vi "handshake_end.vi"(8 "error in (no error)":errorcluster, 11 "server_response (json)":string) -> (0 "error out":errorcluster, 3 "authentication":string)   [LabVIEW 2017, in "rethinkdb.lvlib"]
uses:
  rethinkdb.lvlib
  d907db94-4fb8-4ff2-8f9c-6f68c4a03077.vi
  json_get_names.vi
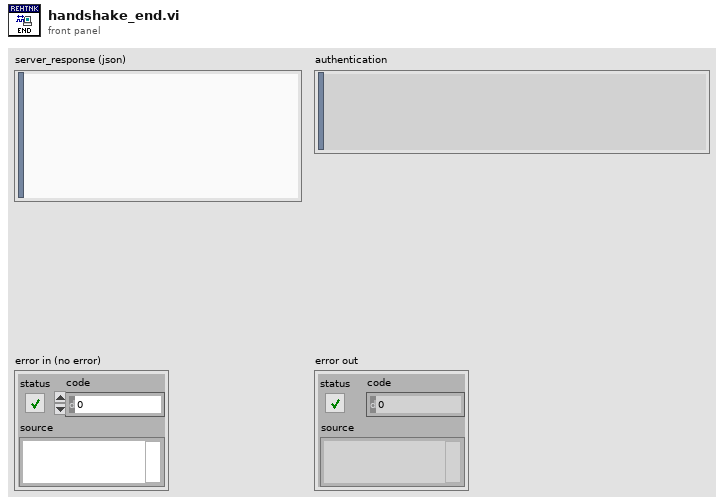
[diagram p1: front panel]
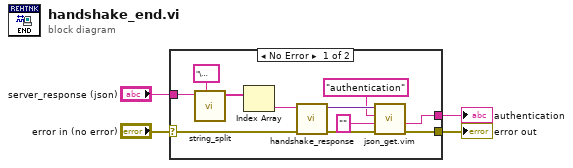
[diagram p0: block diagram]
diagram:
  n1 = case shown="No Error" "error in (no error)" {
    selector: "error in (no error)" -> [w12 w16]
    tunnel: [w7 w16] -> w3
    tunnel: [w6 _] -> w2
    tunnel: "server_response (json)" -> [w13 _]
    frame No Error {
      n2 = call "string_split.vi"("char (0x00)"="\u0000", "data in"=w13) -> ("messages"=w15:string[])  [unwired: 8 in, 1 out]
      n3 = Index Array(array=w15) -> (element=w14:string)  [unwired: 1 in]
      n4 = call "handshake_response.vi"("error in (no error)"=w12, "response"=w14) -> ("error out"=w10:errorcluster, "value"=w9:variant)  [unwired: 8 in]
      n5 = call "json_get.vim"("error in (no error)"=w10, "default"="", "name"="authentication" ("key"), "variant in"=w9) -> ("error out"=w7:errorcluster, "value"=w6:string)  [unwired: 4 in, 2 out]
    }
    frame Error {
    }
  }
  "error out" <- w3
  "authentication" <- w2
